vi "DataSocket-Manager.vi"() -> ()   [LabVIEW 2019]
doc: "Uses DataSocket to write array data. This example works for writing the data to the DataSocket Server (for live data). \n \nThe Writer, Server, and Reader can all be on the same computer or different computers. The Writer and Reader URLs should point to the computer where the DataSocket Server is."
panel:
  out "ProcState":T1(ring)
  # "Overview: Demonstrates the use of the DataSocket functions to manage the remote client works\nRequirements: Windows\nInstructions:\n1. Run the DataSocket Server by navigating the Windows start menu to National Instruments > DataSocket > DataSocket Server.\n2. Run the DataSocket-Manager vi.\n3. Open and run DaraSocket-Client vi.\n4. Checkout the state change in indicator ProcState."
  # "DataSocket - Manager"
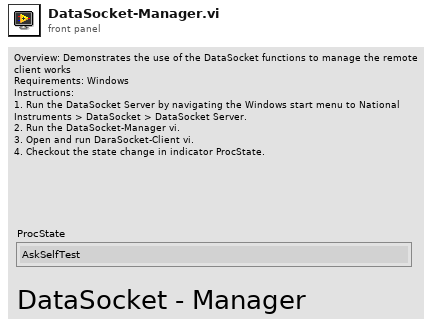
[diagram p1: front panel]
types:
  T1 = enum16{"AskSelfTest", "WaitACK", "StartProc", "EndProc"}
  T2 = enum16{"Read", "Write", "ReadWrite", "BufferedRead", "BufferedReadWrite"}
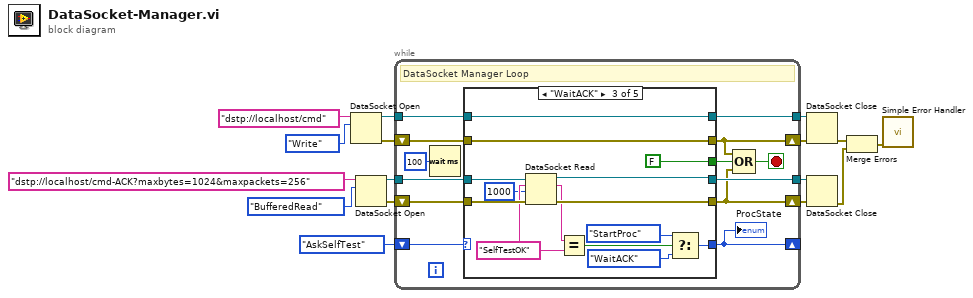
[diagram p0: block diagram]
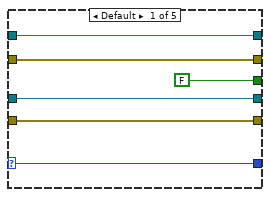
[diagram p2: hidden frame]
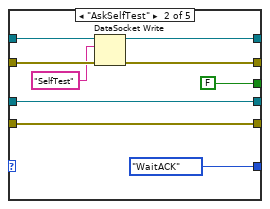
[diagram p3: hidden frame]
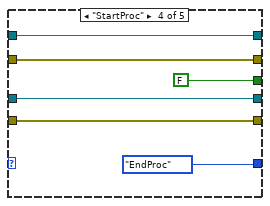
[diagram p4: hidden frame]
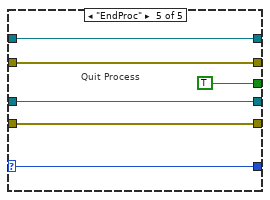
[diagram p5: hidden frame]
diagram:
  n1 = DataSocket Open(10:T2."Write" ("mode"), 11:"dstp://localhost/cmd" ("Write Location")) -> (0:w14:errorcluster, 3:w15:refnum<k13>)  [unwired: 2 in]
  n2 = DataSocket Open(10:T2."BufferedRead" ("mode"), 11:"dstp://localhost/cmd-ACK?maxbytes=1024&maxpackets=256" ("Write Location")) -> (0:w1:errorcluster, 3:w2:refnum<k13>)  [unwired: 2 in]
  n3 = while {
    tunnel: w15 -> [w28]
    tunnel: [w26] -> w13
    tunnel: w2 -> [w24]
    tunnel: [w23] -> w7
    shift-right: [w17] -> _
    shift-left: T1."AskSelfTest" -> [w25]
    shift-right: [w20] -> w16
    shift-left: w14 -> [w29]
    shift-right: [w19] -> w6
    shift-left: w1 -> [w22]
    stop <- w21 stop-if-true
    # "DataSocket Manager Loop"
    n4 = Wait (ms)(milliseconds to wait=u32 100) -> ()  [unwired: 1 out]
    n5 = case shown="\"WaitACK\"" w25 {
      selector: w25 -> [w31 _ _ _ w65]
      tunnel: w29 -> [w34 w44 w51 w63 w69]
      tunnel: w28 -> [w35 w43 w50 w64 w70]
      tunnel: [w34 w41 w51 w63 w69] -> w20
      tunnel: [w35 w40 w50 w64 w70] -> w26
      tunnel: w24 -> [w33 w39 w58 w62 w68]
      tunnel: [w33 w39 w56 w62 w68] -> w23
      tunnel: [w31 T1."WaitACK" w46 T1."EndProc" w65] -> w17
      tunnel: w22 -> [w32 w36 w57 w61 w67]
      tunnel: [w32 w36 w55 w61 w67] -> w19
      tunnel: [FALSE FALSE FALSE FALSE TRUE] -> w18
      frame Default {
      }
      frame "AskSelfTest" {
        n6 = DataSocket Write(8:w44, 10:"SelfTest", 11:w43) -> (0:w41:errorcluster, 3:w40:refnum<k13>)  [unwired: 2 out]
      }
      frame "WaitACK" {
        w53 = "SelfTestOK"
        n7 = DataSocket Read(8:w57, 9:1000 ("ms timeout (10000)"), 10:w53, 11:w58) -> (0:w55:errorcluster, 2:w54:string, 3:w56:refnum<k13>)  [unwired: 1 in, 4 out]
        n8 = Equal?(x=w54, y=w53) -> (x = y?=w49:bool)
        n9 = Select(t=T1."StartProc", s=w49, f=T1."WaitACK") -> (s? t:f=w46:T1)
      }
      frame "StartProc" {
      }
      frame "EndProc" {
        # "Quit Process"
      }
    }
    "ProcState" <- w17
    n10 = Compound Arithmetic op=OR(w20, w18, w19) -> (w21:bool)
  }
  n11 = DataSocket Close(8:w16, 11:w13) -> (0:w4:errorcluster)  [unwired: 1 in, 1 out]
  n12 = DataSocket Close(8:w6, 11:w7) -> (0:w3:errorcluster)  [unwired: 1 in, 1 out]
  n13 = Merge Errors(w4, w3) -> (w5:errorcluster)
  n14 = call <vilib>:"Simple Error Handler.vi"("error in (no error)"=w5) -> ()  [unwired: 4 in, 5 out]
